vi "Determine Value Source.vi"(8 "error in (no error)":errorcluster, 11 "Field Factory in":refnum<class "Field Factory.lvclass">) -> (0 "error out":errorcluster, 2 "Value Source":refnum<class "Value Source.lvclass">, 3 "Field Factory out":refnum<class "Field Factory.lvclass">)   [LabVIEW 2020, in "Composed Fields.lvlib" / "Field Factory.lvclass"]
uses:
  Field Factory.lvclass
  C:/Users/User/Desktop/Raman Program/LV-Database-OOP/source/Database OOP/Column Libraries/Column Configuration/Composed Column Factory.lvclass
  Composed Columns/Value Source Interface Class/Value Source.lvclass
  Basic Fields/Field Configurations/Field Configuration Class/Field Configuration.lvclass
  Column Configuration/Composed Column Factory.lvclass/Composed Column Factory.ctl
  Ctrl Renum Value Source Class/Ctrl Refnum Value Source.lvclass
  C:/Users/User/Desktop/Raman Program/LV-Database-OOP/source/Database OOP/Column Libraries/Composed Columns/Value Source Interface Class/Value Source.lvclass
  Path Refnum/Path Ctrl Refnum.lvclass
  C:/Users/User/Desktop/Raman Program/LV-Database-OOP/source/Database OOP/Column Libraries/Ctrl Renum Value Source Class/Ctrl Refnum Value Source.lvclass
  String Ctrl Refnum Source/String Ctrl Refnum Source.lvclass
  Numeric Ctrl Refnum Source/Numeric Ctrl Refnum Source.lvclass
  Timestamp Ctrl Value Source/Timestamp Ctrl Value Source.lvclass
  Text Ring Ctrl Refnum Source/Text Ring Ctrl Refnum Source.lvclass
  Basic Columns/Column Configuration/Basic Column Configuration Class/Column Configuration.lvclass
  Column Configuration/Composed Column Factory.lvclass
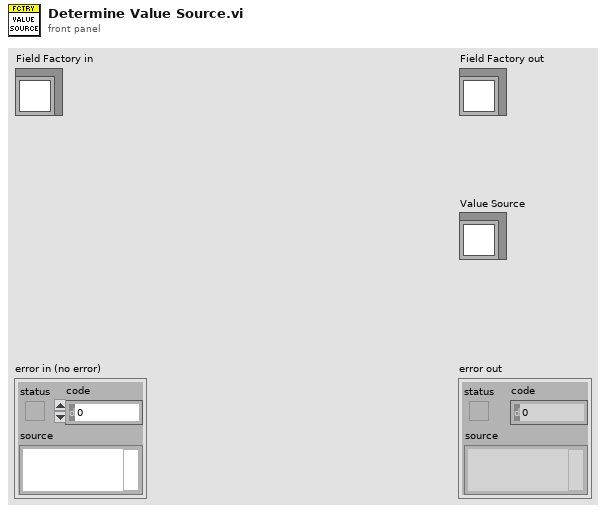
[diagram p1: front panel]
types:
  T1 = typedef "Database Interfaces.lvlib/Database data type.ctl" = enum16{"Undefined", "String", "Long (I32)", "Single (SGL)", "Double (DBL)", "Date/Time", "Binary"}
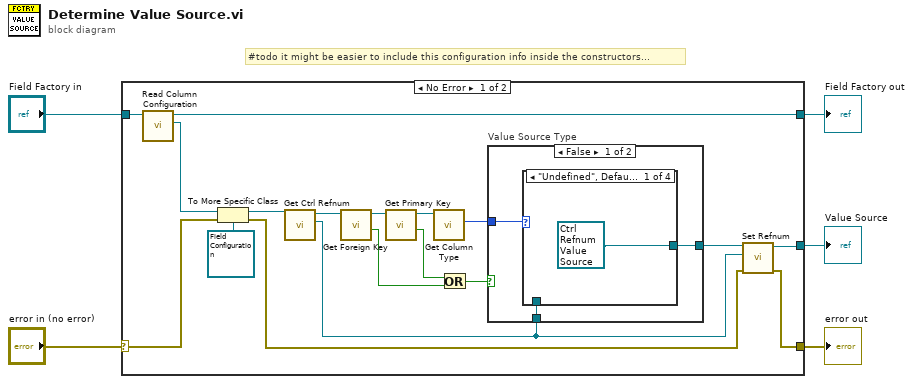
[diagram p0: block diagram]
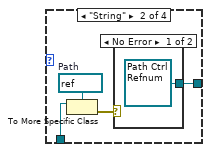
[diagram p2: hidden frame]
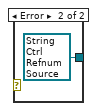
[diagram p3: hidden frame]
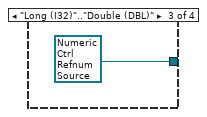
[diagram p4: hidden frame]
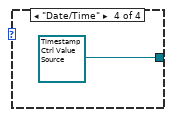
[diagram p5: hidden frame]
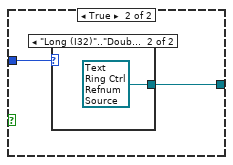
[diagram p6: hidden frame]
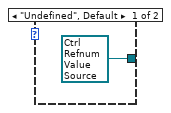
[diagram p7: hidden frame]
diagram:
  # "#todo it might be easier to include this configuration info inside the constructors..."
  n1 = case shown="No Error" "error in (no error)" {
    selector: "error in (no error)" -> [w18 w41]
    tunnel: "Field Factory in" -> [w20 w40]
    tunnel: [w21 w41] -> w3
    tunnel: [w19 w40] -> w2
    tunnel: [w22 _] -> w1
    frame No Error {
      n2 = call "Read Column Configuration.vi"("Composed Column Factory in"=w20) -> ("Column Interfaces.lvlib:Column Configuration.lvclass"=w16:refnum<class "Column Configuration.lvclass">, "Composed Column Factory out"=w19:refnum<class "Field Factory.lvclass">)  [unwired: 8 in, 1 out]
      n3 = To More Specific Class(target class=refnum<class "Field Configuration.lvclass"> refnum ("Field Interfaces.lvlib:Field Configuration.lvclass"), reference=w16, error in=w18) -> (specific class reference=w14:refnum<class "Field Configuration.lvclass">, error out=w15:errorcluster)
      n4 = call-dynamic "Get Ctrl Refnum.vi"("Field Configuration in"=w14) -> ("Ctl Refnum"=w6:refnum<vi>, "Field Configuration out"=w13:refnum<class "Field Configuration.lvclass">)  [unwired: 8 in, 1 out]
      n5 = call-dynamic "Get Foreign Key.vi"("Basic Column Configuration in"=w13) -> ("Is a FK?"=w7:bool, "Basic Column Configuration out"=w11:refnum<class "Field Configuration.lvclass">)  [unwired: 7 in, 2 out]
      n6 = call-dynamic "Get Primary Key.vi"("Basic Column Configuration in"=w11) -> ("Is a PK?"=w8:bool, "Basic Column Configuration out"=w10:refnum<class "Field Configuration.lvclass">)  [unwired: 7 in, 2 out]
      n7 = call-dynamic "Get Column Type.vi"("Basic Column Configuration in"=w10) -> ("Column Type"=w12:T1)  [unwired: 8 in, 2 out]
      n8 = Or(x=w8, y=w7) -> (x .or. y?=w9:bool)
      n9 = case "Value Source Type" shown="False" w9 {
        tunnel: [w25 w36] -> w23
        tunnel: w12 -> [w26 w37]
        tunnel: w6 -> [w24 _]
        frame False {
          n10 = case shown="\"Undefined\", Default" w26 {
            tunnel: [refnum<class "Ctrl Refnum Value Source.lvclass"> refnum ("Composed Columns.lvlib:Ctrl Refnum Value Source.lvclass") w28 refnum<class "Numeric Ctrl Refnum Source.lvclass"> refnum ("Composed Columns.lvlib:Numeric Ctrl Refnum Source.lvclass") refnum<class "Timestamp Ctrl Value Source.lvclass"> refnum ("Composed Columns.lvlib:Timestamp Ctrl Value Source.lvclass")] -> w25
            tunnel: w24 -> [_ w31 _ _]
            frame "Undefined", Default {
            }
            frame "String" {
              w30 = refnum<vi> refnum  # Path
              n11 = To More Specific Class(target class=w30, reference=w31) -> (error out=w29:errorcluster)  [unwired: 1 in, 1 out]
              n12 = case shown="No Error" w29 {
                tunnel: [refnum<class "Path Ctrl Refnum.lvclass"> refnum ("Composed Columns.lvlib:Path Ctrl Refnum.lvclass") refnum<class "String Ctrl Refnum Source.lvclass"> refnum ("Composed Columns.lvlib:String Ctrl Refnum Source.lvclass")] -> w28
                frame No Error {
                }
                frame Error {
                }
              }
            }
            frame "Long (I32)".."Double (DBL)" {
            }
            frame "Date/Time" {
            }
          }
        }
        frame True {
          n13 = case shown="\"Long (I32)\"..\"Double (DBL)\"" w37 {
            tunnel: [refnum<class "Ctrl Refnum Value Source.lvclass"> refnum ("Composed Columns.lvlib:Ctrl Refnum Value Source.lvclass") refnum<class "Text Ring Ctrl Refnum Source.lvclass"> refnum ("Composed Columns.lvlib:Text Ring Ctrl Refnum Source.lvclass")] -> w36
            frame "Undefined", Default {
            }
            frame "Long (I32)".."Double (DBL)" {
            }
          }
        }
      }
      n14 = call "Set Refnum.vi"("error in (no error)"=w15, "Ctl Refnum"=w6, "Ctrl Refnum Value Source in"=w23) -> ("error out"=w21:errorcluster, "Ctrl Refnum Value Source out"=w22:refnum<class "Ctrl Refnum Value Source.lvclass">)  [unwired: 7 in]
    }
    frame Error {
    }
  }
  "error out" <- w3
  "Field Factory out" <- w2
  "Value Source" <- w1
